vi "Draw Collapsed IO.vi"(10 "State":T1, 11 "Picture In":picture) -> (3 "Picture":picture)   [LabVIEW 2020, in "Parallel Diagram Block.xnode"]
uses:
  Parallel Diagram Block.xnode
  Parallel Block/Direction.ctl
  Parallel Block/Parallel Block.lvlib
  Parallel Block/Terminal Mode.ctl
  Parallel Block/Value Type.ctl
  Parallel Block/Type Descriptor.ctl
  <vilib>/picture/picture.llb/imagedata.ctl
  State.ctl
  Parallel Block/Terminal Type.ctl
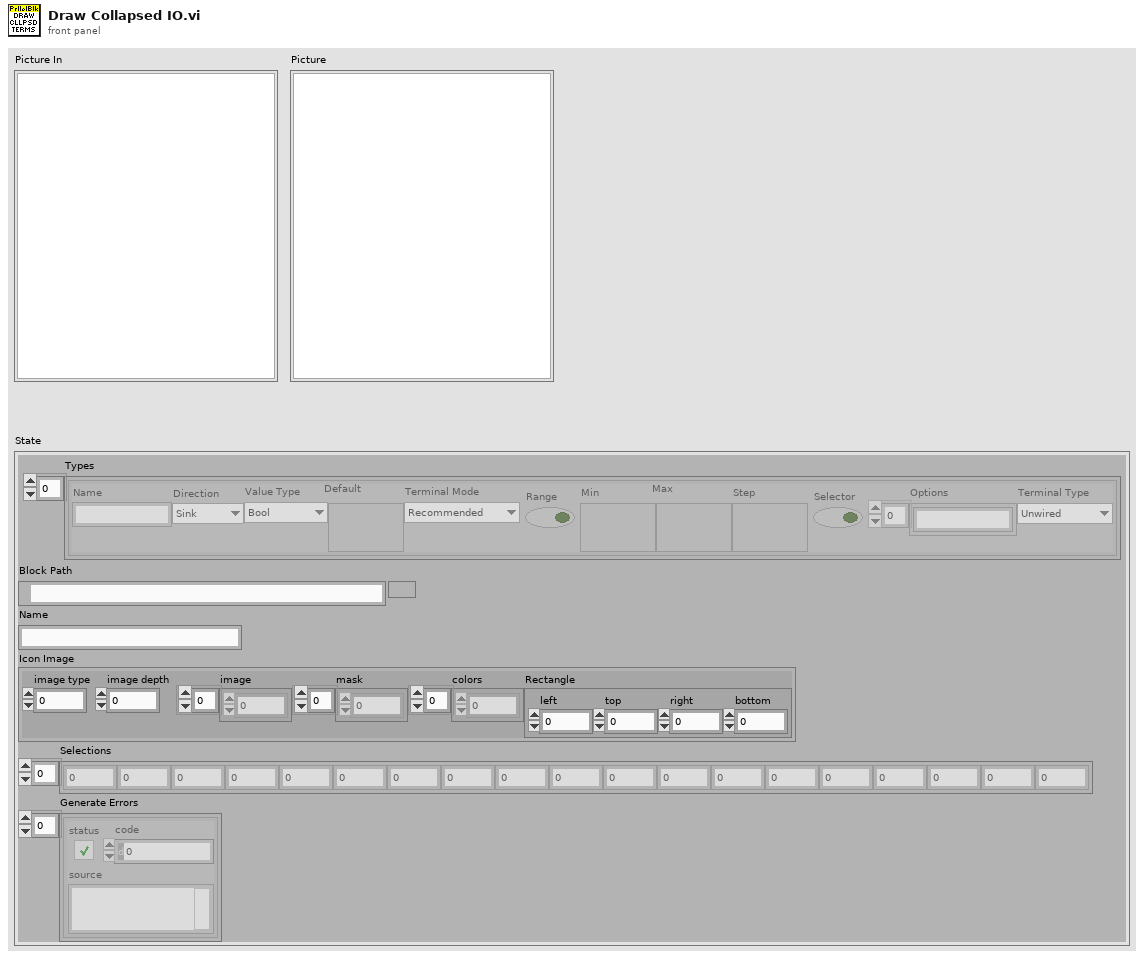
[diagram p1: front panel]
types:
  T1 = typedef "Parallel Diagram Block.xnode/State.ctl" = cluster{"Types":T2[], "Block Path":path, "Name":string, "Icon Image":T7, "Selections":i32[], "Generate Errors":errorcluster[]}
  T2 = typedef "Parallel Block.lvlib/Type Descriptor.ctl" = cluster{"Name":string, "Direction":T3, "Value Type":T4, "Default":variant, "Terminal Mode":T5, "Range":bool, "Min":variant, "Max":variant, "Step":variant, "Selector":bool, "Options":string[], "Terminal Type":T6}
  T3 = typedef "Parallel Block.lvlib/Direction.ctl" = enum16{"Sink", "Source"}
  T4 = typedef "Parallel Block.lvlib/Value Type.ctl" = enum16{"Unknown", "Bool", "U8", "U16", "U32", "U64", "I8", "I16", "I32", "I64", "SGL", "DBL", "CSG", "CDB", "CDBWfm", "String", "DBLWfm"}
  T5 = typedef "Parallel Block.lvlib/Terminal Mode.ctl" = enum16{"Recommended", "Required", "None"}
  T6 = typedef "Parallel Block.lvlib/Terminal Type.ctl" = enum16{"Unwired", "BadType", "Connection", "Value", "Control Ref", "BadRefType"}
  T7 = typedef "imagedata.ctl" = cluster{"image type":i32, "image depth":i32, "image":u8[], "mask":u8[], "colors":u32[], "Rectangle":cluster{"left":i16, "top":i16, "right":i16, "bottom":i16}}
  T8 = cluster{"left":i16, "top":i16, "right":i16, "bottom":i16}
  T9 = typedef "NI_XNodeSupport.lvlib/XNodeRect32.ctl" = cluster{"Left":T10, "Top":T10, "Right":T10, "Bottom":T10}
  T10 = typedef "NI_XNodeSupport.lvlib/XNodeInt.ctl" = i32
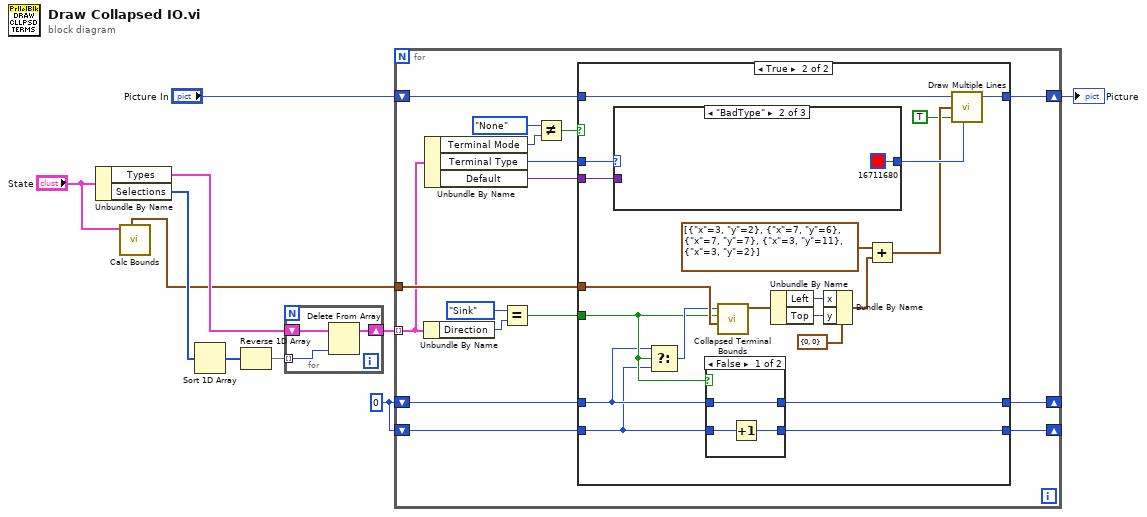
[diagram p0: block diagram]
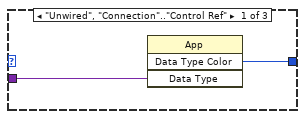
[diagram p3: hidden frame]
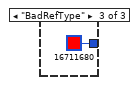
[diagram p4: hidden frame]
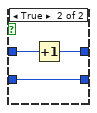
[diagram p5: hidden frame]
diagram:
  w2 = 0
  n1 = Unbundle By Name("State") -> ("Types"=w3:T2[], "Selections"=w6:i32[])
  n2 = call "Calc Bounds.vi"("State"="State") -> ("Full Bounds"=w1:T8)  [unwired: 6 in, 4 out]
  n3 = Sort 1D Array(array=w6) -> (sorted array=w5:i32[])
  n4 = Reverse 1D Array(array=w5) -> (reversed array=w4:i32[])
  n5 = for {
    tunnel: w4 -> [w12] mode=indexing
    shift-right: [w13] -> w10
    shift-left: w3 -> [w11]
    n6 = Delete From Array(array=w11, index=w12) -> (array with subset deleted=w13:T2[])  [unwired: 1 in, 1 out]
  }
  n7 = for {
    tunnel: w10 -> [w23] mode=indexing
    shift-right: [w26] -> w8
    shift-left: "Picture In" -> [w27]
    tunnel: w1 -> [w25]
    shift-right: [w19] -> _
    shift-left: w2 -> [w21]
    shift-right: [w18] -> _
    shift-left: w2 -> [w20]
    n8 = Unbundle By Name(w23) -> ("Direction"=w24:T3)
    n9 = Unbundle By Name(w23) -> ("Terminal Mode"=w17:T5, "Terminal Type"=w14:T6, "Default"=w28:variant)
    n10 = Equal?(x=Direction."Sink", y=w24) -> (x = y?=w22:bool)
    n11 = Not Equal?(x=Terminal_Mode."None", y=w17) -> (x != y?=w15:bool)
    n12 = case shown="True" w15 {
      tunnel: w28 -> [_ w52]
      tunnel: w27 -> [w32 w51]
      tunnel: [w32 w50] -> w26
      tunnel: w25 -> [_ w48]
      tunnel: w22 -> [_ w39]
      tunnel: w21 -> [w31 w38]
      tunnel: w20 -> [w30 w37]
      tunnel: [w31 w36] -> w19
      tunnel: [w30 w35] -> w18
      tunnel: w14 -> [_ w33]
      frame False {
      }
      frame True {
        n13 = case shown="\"BadType\"" w33 {
          tunnel: w52 -> [w54 _ _]
          tunnel: [w53 u32 16711680 ("Data Type Color") u32 16711680 ("Data Type Color")] -> w49
          frame "Unwired", "Connection".."Control Ref" {
            n14 = invoke class="App" method="Data Type Color"("Data Type"=w54) -> ("Data Type Color"=w53:u32)  [unwired: 3 in, 3 out]
          }
          frame "BadType" {
          }
          frame "BadRefType" {
          }
        }
        n15 = Select(t=w38, s=w39, f=w37) -> (s? t:f=w40:i32)
        n16 = case shown="False" w39 {
          tunnel: w38 -> [w57 w62]
          tunnel: w37 -> [w59 w60]
          tunnel: [w57 w61] -> w36
          tunnel: [w58 w60] -> w35
          frame False {
            n17 = Increment(x=w59) -> (x+1=w58:i32)
          }
          frame True {
            n18 = Increment(x=w62) -> (x+1=w61:i32)
          }
        }
        n19 = call "Collapsed Terminal Bounds.vi"("Border Without Terminals"=w48, "Input"=w39, "Index"=w40) -> ("Bounds"=w47:T9)  [unwired: 8 in]
        n20 = Unbundle By Name(w47) -> ("Left"=w45:T10, "Top"=w44:T10)
        n21 = Bundle By Name(cluster=cluster{"x":i32, "y":i32} {"x"=0, "y"=0}, "x"=w45, "y"=w44) -> (w42:cluster{"x":i32, "y":i32})
        n22 = Add(x=cluster{"x":i16, "y":i16}[] [{"x"=3, "y"=2}, {"x"=7, "y"=6}, {"x"=7, "y"=7}, {"x"=3, "y"=11}, {"x"=3, "y"=2}] ("line endpoints"), y=w42) -> (x+y=w41:cluster{"x":i32, "y":i32}[])
        n23 = call <vilib>:"Draw Multiple Lines.vi"("picture"=w51, "line endpoints"=w41, "fill?(F)"=TRUE, "color(black)"=w49) -> ("new picture"=w50:picture)  [unwired: 5 in]
      }
    }
  }
  "Picture" <- w8
